vi "Example.vi"() -> ()   [LabVIEW 2015, in "CR5.lvclass"]
uses:
  CR5.lvclass
  <vilib>/Platform/TimedLoop/XDataNode/XDataNode.xnode
  <vilib>/Platform/TimedLoop/XDataNode/nitl_modes.ctl
  <vilib>/Platform/TimedLoop/XDataNode/XDNodeRunTimeDep.lvlib
  <vilib>/Platform/TimedLoop/XDataNode/wakeup.ctl
  <vilib>/Platform/TimedLoop/XDataNode/timing_clust.ctl
  <userlib>/_Session Fwk/Session - Root.lvclass
  Reusable/Session APIs/File Access/Config Data/Config Data.lvclass
  Reusable/Session Log/System Log.lvclass
  Reusable/Session APIs/Serial/Serial Session.lvclass
panel:
  in  "Main Path":path
  in  "Cfg Path":path
  in  "Stop":bool
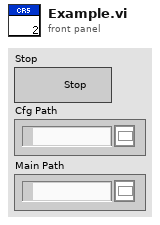
[diagram p1: front panel]
types:
  T1 = typedef "Session - Root.lvclass/Session Handle.ctl" = refnum<data-value>
  T2 = typedef "XDNodeRunTimeDep.lvlib/timing_clust.ctl" = cluster{"Expected End [f-1]":u64, "Actual End [f-1]":u64, "Finished Late? [f-1]":bool, "Expected End [i-1]":u64, "Actual End [i-1]":u64, "Finished Late? [i-1]":bool, "Expected Start [i]":u64, "Actual Start [i]":u64, "Expected Start [f]":u64, "Actual Start [f]":u64, "Source Name":string, "Structure Name":string, "Period":i64, "Deadline":i64, "Offset":i64, "Start":i64, "Priority":i32, "Timeout":i32, "Mode":T3, "Wakeup Reason":T4, "Error":errorcluster, "Source Type":string, "Secondary Source Type":string, "Global End Time":u64, "Global Start Time":u64, "Frame Duration":u64, "Iteration Duration":u64, "Assigned CPU":i32, "I/O Scan Engine Mode":u32}
  T3 = typedef "XDNodeRunTimeDep.lvlib/nitl_modes.ctl" = enum32{"No Change", "Process missed periods, maintain original phase", "Discard missed periods, maintain original phase", "Process missed periods, ignore original phase", "Discard missed periods, ignore original phase"}
  T4 = typedef "XDNodeRunTimeDep.lvlib/wakeup.ctl" = enum32{"Normal", "Aborted", "Asynchronous wakeup", "Timing source error", "Timed loop error", "Timeout"}
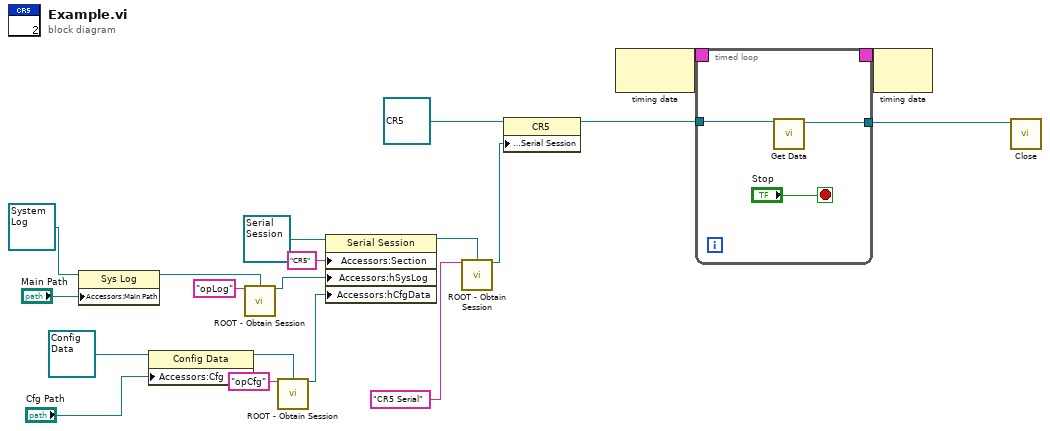
[diagram p0: block diagram]
diagram:
  n1 = property class="Sys Log"(reference=refnum<class "System Log.lvclass"> refnum ("Sys Log"), "Accessors:Main Path"="Main Path") -> (reference out=w9:refnum<class "System Log.lvclass">)  [unwired: 1 in, 1 out]
  n2 = property class="Config Data"(reference=refnum<class "Config Data.lvclass"> refnum ("Config Data"), "Accessors:Cfg Path"="Cfg Path") -> (reference out=w14:refnum<class "Config Data.lvclass">)  [unwired: 1 in, 1 out]
  n3 = call <userlib>:"ROOT - Obtain Session.vi"("Session Name ()"="opLog", "OBJ - Session"=w9) -> ("Session Handle"=w8:T1)  [unwired: 11 in, 2 out]
  n4 = call <userlib>:"ROOT - Obtain Session.vi"("Session Name ()"="opCfg", "OBJ - Session"=w14) -> ("Session Handle"=w12:T1)  [unwired: 11 in, 2 out]
  n5 = property class="Serial Session"(reference=refnum<class "Serial Session.lvclass"> refnum ("Serial Session"), "Accessors:Section"="CR5" ("Section"), "Accessors:hSysLog"=w8, "Accessors:hCfgData"=w12) -> (reference out=w5:refnum<class "Serial Session.lvclass">)  [unwired: 1 in, 1 out]
  n6 = call <userlib>:"ROOT - Obtain Session.vi"("Session Name ()"="CR5 Serial", "OBJ - Session"=w5) -> ("Session Handle"=w4:T1)  [unwired: 11 in, 2 out]
  n7 = property class="CR5"(reference=refnum<class "CR5.lvclass"> refnum ("CR5.lvclass"), "Accessors:Serial Session"=w4) -> (reference out=w3:refnum<class "CR5.lvclass">)  [unwired: 1 in, 1 out]
  n8 = node-c288() -> (w20:T2)  [unwired: 1 in]
  n9 = timed-loop {
    timing: w20 -> [_]
    timing-out: [_] -> w19
    tunnel: w3 -> [w22]
    tunnel: [w21] -> w1
    stop <- "Stop" stop-if-true
    n10 = call "Get Data.vi"("CR5 in"=w22) -> ("CR5 out"=w21:refnum<class "CR5.lvclass">)  [unwired: 8 in, 2 out]
  }
  n11 = node-c288(w19) -> ()  [unwired: 1 out]
  n12 = call-dynamic "Close.vi"("CR5 in"=w1) -> ()  [unwired: 9 in, 2 out]
